vi "Read Subscriber ID.vi"(8 "error in (no error)":errorcluster, 11 "Subscriber in":refnum<class "Subscriber.lvclass">) -> (0 "error out":errorcluster, 2 "Subscriber ID":i64, 3 "Subscriber out":refnum<class "Subscriber.lvclass">)   [LabVIEW 2024, in "Subscriber.lvclass"]
uses:
  Subscriber.lvclass
  Subscriber.lvclass/Subscriber.ctl
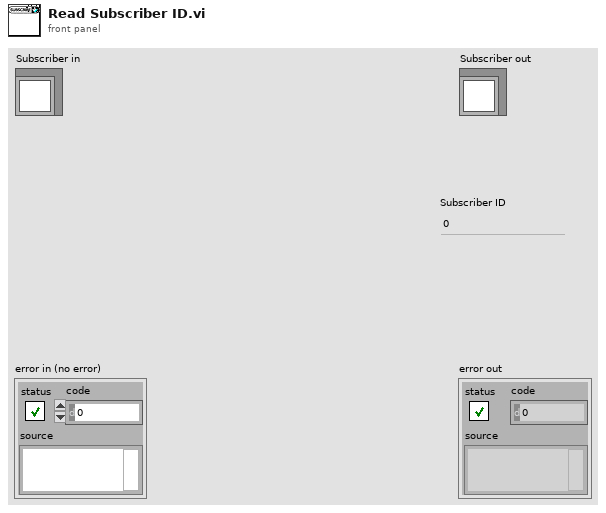
[diagram p1: front panel]
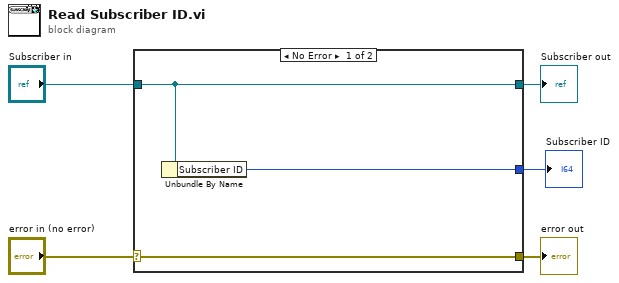
[diagram p0: block diagram]
diagram:
  n1 = case shown="No Error" "error in (no error)" {
    selector: "error in (no error)" -> [w8 w9]
    tunnel: [w8 w9] -> w4
    tunnel: [w7 w10] -> w2
    tunnel: "Subscriber in" -> [w7 w10]
    tunnel: [w6 _] -> w1
    frame No Error {
      n2 = Unbundle By Name(w7) -> ("Subscriber ID"=w6:i64)
    }
    frame Error {
    }
  }
  "error out" <- w4
  "Subscriber out" <- w2
  "Subscriber ID" <- w1
